vi "Create.vi"(10 "Position":T1) -> (3 "Particle out":refnum<class "Particle.lvclass">)   [LabVIEW 2020, in "Particle.lvclass"]
uses:
  Particle.lvclass
  Particle/Position.ctl
  Particle.lvclass/Particle.ctl
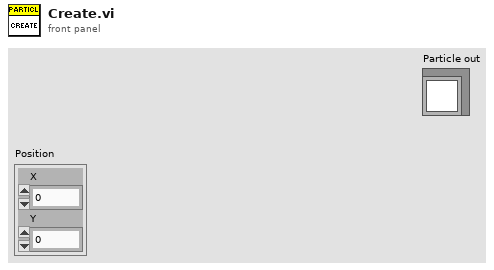
[diagram p1: front panel]
types:
  T1 = typedef "Particle.lvclass/Position.ctl" = cluster{"X":i32, "Y":i32}
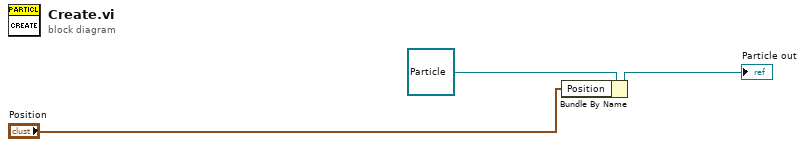
[diagram p0: block diagram]
diagram:
  n1 = Bundle By Name(cluster=refnum<class "Particle.lvclass"> refnum ("Particle out"), "Position"="Position") -> (→"Particle out":refnum<class "Particle.lvclass">)
